vi "XY点至极坐标点和复数点(2D）.vi"(8 "Error In":errorcluster caption="错误输入", 11 "点":T2[][](array[typedef])) -> (0 "Error Out":errorcluster caption="错误输出", 2 "复数点":cdb[][](array[numeric]), 3 "极坐标点":T1[][](array[typedef]))   [LabVIEW 2012, in "几何工具.lvlib"]
uses:
  <vilib>/Utility/miscctls.llb/LVPointDoubleTypeDef.ctl
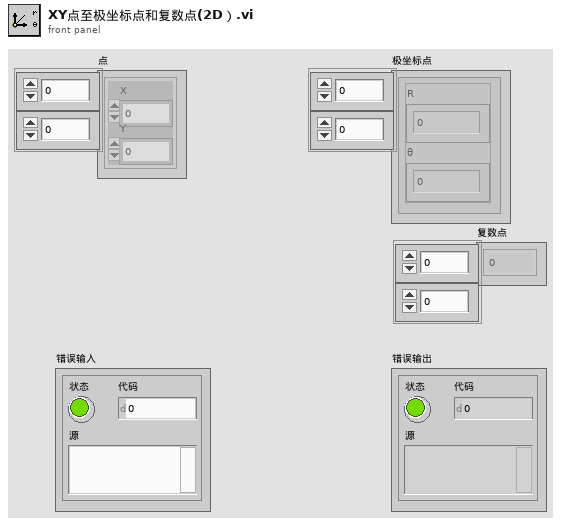
[diagram p1: front panel]
types:
  T1 = typedef "几何工具.lvlib/极坐标.ctl" = cluster{"R":dbl, "θ":dbl}
  T2 = typedef "LVPointDoubleTypeDef.ctl" = cluster{"X":dbl, "Y":dbl}
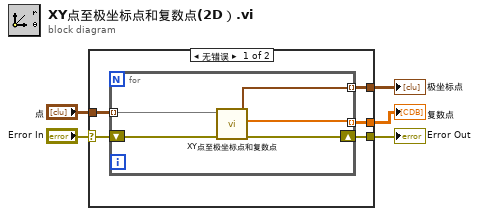
[diagram p0: block diagram]
diagram:
  n1 = case shown="无错误" "Error In" {
    selector: "Error In" -> [w9 w16]
    tunnel: [w8 w16] -> w4
    tunnel: "点" -> [w10 _]
    tunnel: [w7 _] -> w2
    tunnel: [w6 _] -> w1
    frame No Error {
      n2 = for {
        tunnel: w10 -> [w15] mode=indexing
        tunnel: [w12] -> w7 mode=indexing
        tunnel: [w11] -> w6 mode=indexing
        shift-right: [w13] -> w8
        shift-left: w9 -> [w14]
        n3 = call-poly "XY点至极坐标点和复数点.vi"("Error In"=w14, "点"=w15) -> ("Error Out"=w13:errorcluster, "复数点"=w11:cdb[], "极坐标点"=w12:T1[])  [unwired: 7 in]
      }
    }
    frame Error {
    }
  }
  "Error Out" <- w4
  "极坐标点" <- w2
  "复数点" <- w1
